vi "Start.vi"(8 "Error In":errorcluster) -> (0 "Error Out":errorcluster)   [LabVIEW 2014, in "Logger.lvlib"]
uses:
  Logger.lvlib
  Run.vi
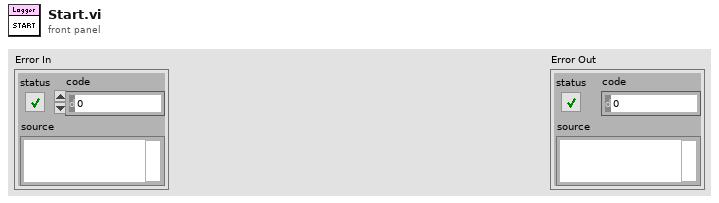
[diagram p1: front panel]
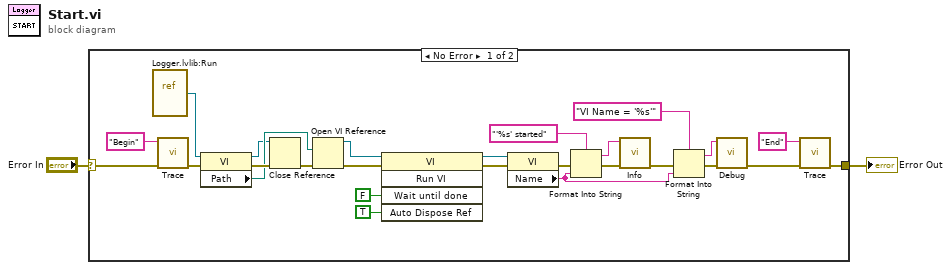
[diagram p0: block diagram]
diagram:
  n1 = case shown="No Error" "Error In" {
    selector: "Error In" -> [w14 w29]
    tunnel: [w11 w29] -> w1
    frame No Error {
      n2 = vi-ref "Logger.lvlib:Run.vi"() -> (w26:refnum<vi>)
      n3 = call "Trace.vi"("Error In"=w14, "Text"="Begin") -> ("Error Out"=w13:errorcluster)  [unwired: 9 in]
      n4 = property class="VI"(reference=w26, error in=w13) -> (reference out=w22:refnum<vi>, error out=w28:errorcluster, "Path"=w27:path)
      n5 = Close Reference(reference=w22, error in (no error)=w28) -> (error out=w23:errorcluster)
      n6 = Open VI Reference(vi path=w27, error in (no error)=w23) -> (vi reference=w3:refnum<vi>, error out=w4:errorcluster)  [unwired: 4 in]
      n7 = invoke class="VI" method="Run VI"(reference=w3, error in=w4, "Wait until done"=FALSE ("Wait Until Done"), "Auto Dispose Ref"=TRUE ("Auto Dispose Reference")) -> (reference out=w19:refnum<vi>, error out=w21:errorcluster)  [unwired: 1 in, 3 out]
      n8 = property class="VI"(reference=w19, error in=w21) -> (error out=w20:errorcluster, "Name"=w16:string)  [unwired: 1 out]
      n9 = Format Into String(format string="'%s' started", error in=w20, w16) -> (resulting string=w8:string, error out=w10:errorcluster)  [unwired: 1 in]
      n10 = call "Info.vi"("Error In"=w10, "Text"=w8) -> ("Error Out"=w9:errorcluster)  [unwired: 9 in]
      n11 = Format Into String(format string="VI Name = '%s'", error in=w9, w16) -> (resulting string=w5:string, error out=w7:errorcluster)  [unwired: 1 in]
      n12 = call "Debug.vi"("Error In"=w7, "Text"=w5) -> ("Error Out"=w6:errorcluster)  [unwired: 9 in]
      n13 = call "Trace.vi"("Error In"=w6, "Text"="End") -> ("Error Out"=w11:errorcluster)  [unwired: 9 in]
    }
    frame Error {
    }
  }
  "Error Out" <- w1
